vi "Add new entry.vi"(8 "error in (no error)":errorcluster, 9 "Severity":string="Error", 10 "Text to log":string, 11 "Logbook in":refnum<class "Logbook.lvclass">) -> (0 "error out":errorcluster, 3 "Logbook out":refnum<class "Logbook.lvclass">)   [LabVIEW 2014, in "Logbook.lvclass"]
uses:
  Logbook.lvclass
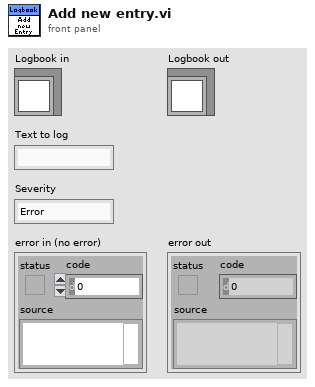
[diagram p1: front panel]
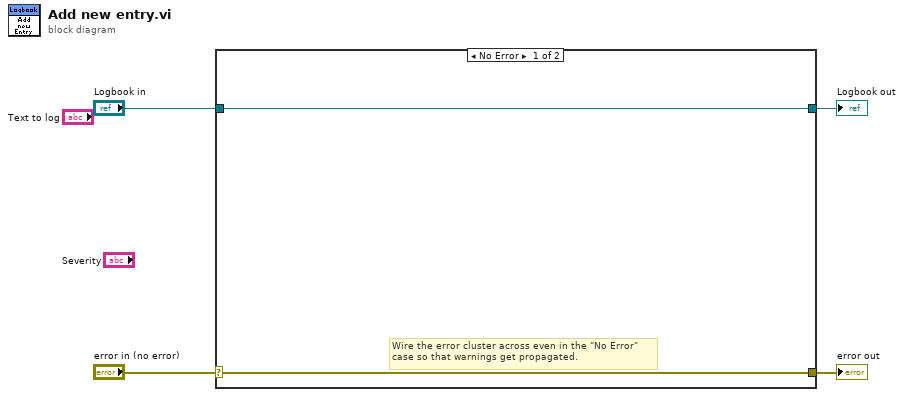
[diagram p0: block diagram]
diagram:
  n1 = case shown="No Error" "error in (no error)" {
    selector: "error in (no error)" -> [w5 w8]
    tunnel: [w5 w8] -> w3
    tunnel: [w6 w7] -> w1
    tunnel: "Logbook in" -> [w6 w7]
    frame No Error {
      # "Wire the error cluster across even in the \"No Error\"\ncase so that warnings get propagated."
    }
    frame Error {
    }
  }
  "error out" <- w3
  "Logbook out" <- w1
